vi "PID Climb (Arms Up).vi"(8 "R Sensor Position":dbl, 11 "L Sensor Position":dbl) -> (0 "R Motor Output":dbl format="%.2f", 3 "L Motor Output":dbl format="%.2f")   [LabVIEW 2019]
uses:
  <vilib>/addons/control/pid/pid.llb/PID (DBL).vi
  <vilib>/addons/control/pid/NI_PID_pid.lvlib
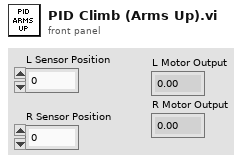
[diagram p1: front panel]
types:
  T1 = cluster{"proportional gain (Kc)":dbl, "integral time (Ti, min)":dbl, "derivative time (Td, min)":dbl}
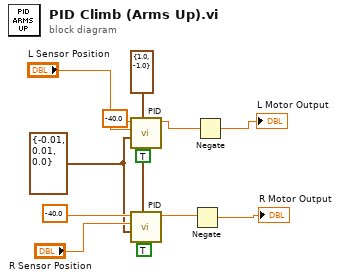
[diagram p0: block diagram]
diagram:
  w5 = T1 {"proportional gain (Kc)"=-0.01, "integral time (Ti, min)"=0.01, "derivative time (Td, min)"=0.0} ("PID gains")
  w10 = cluster{"output high":dbl, "output low":dbl} {"output high"=1.0, "output low"=-1.0} ("output range")
  n1 = call-poly <vilib>:"PID.vi"("reinitialize? (F)"=TRUE, "output range"=w10, "PID gains"=w5, "process variable"="L Sensor Position", "setpoint"=-40.0) -> ("output"=w4:dbl)  [unwired: 5 in, 1 out]
  n2 = call-poly <vilib>:"PID.vi"("reinitialize? (F)"=TRUE, "output range"=w10, "PID gains"=w5, "process variable"="R Sensor Position", "setpoint"=-40.0) -> ("output"=w2:dbl)  [unwired: 5 in, 1 out]
  n3 = Negate(x=w2) -> (-x=→"R Motor Output":dbl)
  n4 = Negate(x=w4) -> (-x=→"L Motor Output":dbl)
